vi "Cache.Result.GetIdx.vi"(11 "String":string="TS[%d].TV[%d].result") -> (1 "TV idx":i32, 2 "TS idx":i32, 3 "remaining string":string="TS[%d].TV[%d].result")   [LabVIEW 2016]
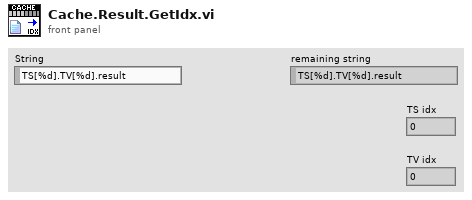
[diagram p1: front panel]
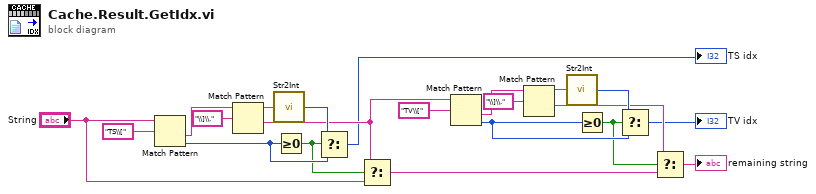
[diagram p0: block diagram]
diagram:
  n1 = Match Pattern(string="String", regular expression="TS\\[") -> (after substring=w15:string, offset past match=w18:i32)  [unwired: 1 in, 2 out]
  n2 = Match Pattern(string=w15, regular expression="\\]\\.") -> (before substring=w9:string, after substring=w12:string)  [unwired: 1 in, 2 out]
  n3 = call "Str2Int.vi"("string"=w9) -> ("Numeric"=w19:i32)
  n4 = Greater Or Equal To 0?(x=w18) -> (x >= 0?=w13:bool)
  n5 = Select(t=w19, s=w13, f=w18) -> (s? t:f=→"TS idx":i32)
  n6 = Select(t=w12, s=w13, f="String") -> (s? t:f=w5:string)
  n7 = Match Pattern(string=w12, regular expression="TV\\[") -> (after substring=w10:string, offset past match=w16:i32)  [unwired: 1 in, 2 out]
  n8 = Match Pattern(string=w10, regular expression="\\]\\.") -> (before substring=w8:string, after substring=w7:string)  [unwired: 1 in, 2 out]
  n9 = call "Str2Int.vi"("string"=w8) -> ("Numeric"=w17:i32)
  n10 = Greater Or Equal To 0?(x=w16) -> (x >= 0?=w6:bool)
  n11 = Select(t=w17, s=w6, f=w16) -> (s? t:f=→"TV idx":i32)
  n12 = Select(t=w7, s=w6, f=w5) -> (s? t:f=→"remaining string":string)
